vi "SetDebugStateOfUMLVIs.vi"() -> ()   [LabVIEW 2016]
panel:
  out "Progress":u8(slide) scale=0.0..100.0
  in  "Debug State for UML VIs":bool
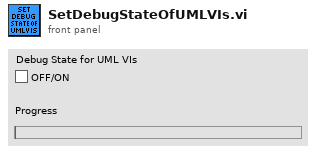
[diagram p1: front panel]
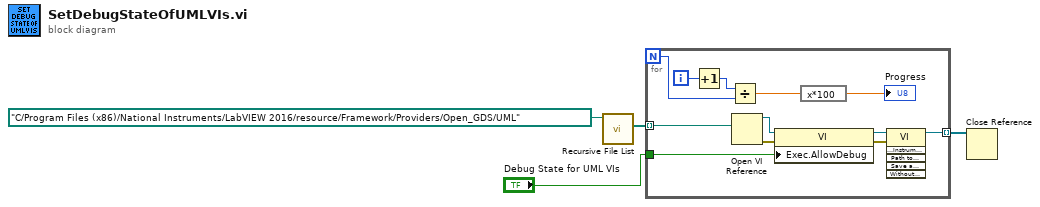
[diagram p0: block diagram]
diagram:
  n1 = call <vilib>:"Recursive File List.vi"("Folder Path"=path "C:/Program Files (x86)/National Instruments/LabVIEW 2016/resource/Framework/Providers/Open_GDS/UML") -> ("All Files in Dir"=w3:path[])  [unwired: 6 in, 4 out]
  n2 = for {
    N -> [w7]
    tunnel: w3 -> [w16] mode=indexing
    tunnel: "Debug State for UML VIs" -> [w14]
    tunnel: [w10] -> w1 mode=indexing
    i -> [w9]
    n3 = Increment(x=w9) -> (x+1=w8:i32)
    n4 = Divide(x=w8, y=w7) -> (x/y=w6:dbl)
    n5 = Open VI Reference(vi path=w16) -> (vi reference=w15:refnum<vi>, error out=w11:errorcluster)  [unwired: 5 in]
    n6 = property class="VI"(reference=w15, error in=w11, "Exec.AllowDebug"=w14) -> (reference out=w13:refnum<vi>, error out=w12:errorcluster)
    n7 = expression code="x*100"(w6) -> (→"Progress":dbl)
    n8 = invoke class="VI" method="Save.Instrument"(reference=w13, error in=w12) -> (reference out=w10:refnum<vi>)  [unwired: 4 in, 5 out]
  }
  n9 = Close Reference(reference=w1) -> ()  [unwired: 1 in, 1 out]
